vi "calc-total-kinetics.vi"(6 "cluster in":T1={"Kinetics"=[], "Spectrum"=[], "Experiments groups"=[], "GRAPH EXPERIMENTAL DATA"=[], "error out"={"status"=FALSE, "code"=0, "source"=""}, "group"=0, "exp selected"=0, "# exp"=0, "kinetics plot names"=[], "spectra plot names"=[], "FromToWave"={"FromWave"=0.0, "ToWave"=0.0}, "Laser shutter task"="", "Accelerator task"="", "Motor task"="", "GRAPH EXPERIMENTAL DATA ref"=refnum, "timedelays"=[0.0, 0.0, 0.0, 0.0, 0.0, 0.0, 0.0, 0.06019061100911815, 0.0521779104562645, 0.045231877429679615, 0.03921051490799832, 0.033990728811568754, 0.029465811603150715, 0.025543260876973825, 0.02214288834180205, 0.01919518054014414, 0.016639877791965713, 0.014424742312398925, 0.012504490320209958, 0.010839866306230088, 0.009396840537117498, 0.008145913389103785, 0.00706151229029317, 0.006121468943269439, 0.005306566140927374, 0.004600144911132549, 0.003987763959109073, 0.0034569044455719407, 0.00299671406541447, 0.0025977851951783253, 0.0022519625739982996, 0.00195217658646366, 0.0016922987392150965, 0.0014670163768006634, 0.0012717240756200802, 0.0011024294957352762, 0.0009556717658856477, 0.0008284507332614981, 0.0007181656316962257, 0.0006225619144775864, 0.0005396851648867825, 0.00046784114226338394, 0.0004055611468220084, 0.0003515719951773376, 0.00030476999279031153, 0.00026419837125694315, 0.00022902772919263772, 0.0001985390768670671, 0.0001721091379728629, 0.00014919760805372974, 0.00012933610911736794], "wavelengths"=[0.0, 0.0, 0.0, 0.0, 0.0, 0.0, 0.0, 0.06019061100911815, 0.0521779104562645, 0.045231877429679615, 0.03921051490799832, 0.033990728811568754, 0.029465811603150715, 0.025543260876973825, 0.02214288834180205, 0.01919518054014414, 0.016639877791965713, 0.014424742312398925, 0.012504490320209958, 0.010839866306230088, 0.009396840537117498, 0.008145913389103785, 0.00706151229029317, 0.006121468943269439, 0.005306566140927374, 0.004600144911132549, 0.003987763959109073, 0.0034569044455719407, 0.00299671406541447, 0.0025977851951783253, 0.0022519625739982996, 0.00195217658646366, 0.0016922987392150965, 0.0014670163768006634, 0.0012717240756200802, 0.0011024294957352762, 0.0009556717658856477, 0.0008284507332614981, 0.0007181656316962257, 0.0006225619144775864, 0.0005396851648867825, 0.00046784114226338394, 0.0004055611468220084, 0.0003515719951773376, 0.00030476999279031153, 0.00026419837125694315, 0.00022902772919263772, 0.0001985390768670671, 0.0001721091379728629, 0.00014919760805372974, 0.00012933610911736794], "Experiment"=refnum, "Commentaires exp"=refnum, "FromToDelay"={"FromDelay"=0.0, "ToDelay"=0.0}}, 7 "delay0":dbl, 8 "# points":i32, 9 "deltaT":dbl) -> (0 "cluster out":T1={"Kinetics"=[], "Spectrum"=[], "Experiments groups"=[], "GRAPH EXPERIMENTAL DATA"=[], "error out"={"status"=FALSE, "code"=0, "source"=""}, "group"=0, "exp selected"=0, "# exp"=0, "kinetics plot names"=[], "spectra plot names"=[], "FromToWave"={"FromWave"=0.0, "ToWave"=0.0}, "Laser shutter task"="", "Accelerator task"="", "Motor task"="", "GRAPH EXPERIMENTAL DATA ref"=refnum, "timedelays"=[0.0, 0.0, 0.0, 0.0, 0.0, 0.0, 0.0, 0.06019061100911815, 0.0521779104562645, 0.045231877429679615, 0.03921051490799832, 0.033990728811568754, 0.029465811603150715, 0.025543260876973825, 0.02214288834180205, 0.01919518054014414, 0.016639877791965713, 0.014424742312398925, 0.012504490320209958, 0.010839866306230088, 0.009396840537117498, 0.008145913389103785, 0.00706151229029317, 0.006121468943269439, 0.005306566140927374, 0.004600144911132549, 0.003987763959109073, 0.0034569044455719407, 0.00299671406541447, 0.0025977851951783253, 0.0022519625739982996, 0.00195217658646366, 0.0016922987392150965, 0.0014670163768006634, 0.0012717240756200802, 0.0011024294957352762, 0.0009556717658856477, 0.0008284507332614981, 0.0007181656316962257, 0.0006225619144775864, 0.0005396851648867825, 0.00046784114226338394, 0.0004055611468220084, 0.0003515719951773376, 0.00030476999279031153, 0.00026419837125694315, 0.00022902772919263772, 0.0001985390768670671, 0.0001721091379728629, 0.00014919760805372974, 0.00012933610911736794], "wavelengths"=[0.0, 0.0, 0.0, 0.0, 0.0, 0.0, 0.0, 0.06019061100911815, 0.0521779104562645, 0.045231877429679615, 0.03921051490799832, 0.033990728811568754, 0.029465811603150715, 0.025543260876973825, 0.02214288834180205, 0.01919518054014414, 0.016639877791965713, 0.014424742312398925, 0.012504490320209958, 0.010839866306230088, 0.009396840537117498, 0.008145913389103785, 0.00706151229029317, 0.006121468943269439, 0.005306566140927374, 0.004600144911132549, 0.003987763959109073, 0.0034569044455719407, 0.00299671406541447, 0.0025977851951783253, 0.0022519625739982996, 0.00195217658646366, 0.0016922987392150965, 0.0014670163768006634, 0.0012717240756200802, 0.0011024294957352762, 0.0009556717658856477, 0.0008284507332614981, 0.0007181656316962257, 0.0006225619144775864, 0.0005396851648867825, 0.00046784114226338394, 0.0004055611468220084, 0.0003515719951773376, 0.00030476999279031153, 0.00026419837125694315, 0.00022902772919263772, 0.0001985390768670671, 0.0001721091379728629, 0.00014919760805372974, 0.00012933610911736794], "Experiment"=refnum, "Commentaires exp"=refnum, "FromToDelay"={"FromDelay"=0.0, "ToDelay"=0.0}}, 1 "Real delay time, ps":dbl=3790.0, 2 "Kinetics, ps":dbl, 3 "Total, ps":dbl, 5 "# points out":i32)   [LabVIEW 2015]
uses:
  controls/control-cluster.ctl
  Classes/Experiments_group.lvclass
  Classes/Experiment.lvclass
panel:
  in  "y":dbl=9000.0 format="%#_13g"
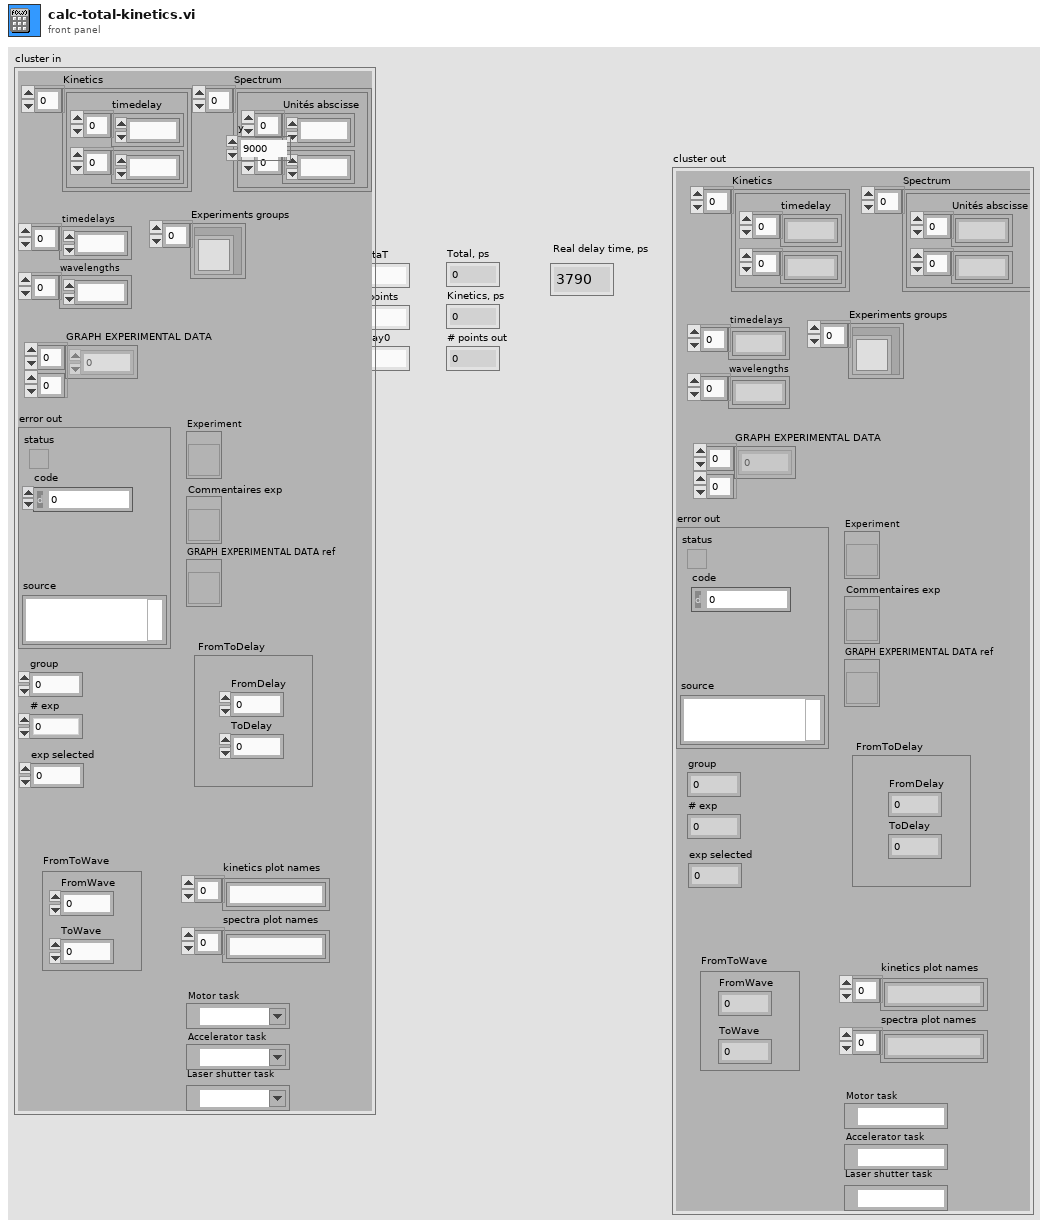
[diagram p1: front panel]
types:
  T1 = typedef "control-cluster.ctl" = cluster{"Kinetics":cluster{"timedelay":dbl[], dbl[]}[], "Spectrum":cluster{"Unités abscisse":dbl[], dbl[]}[], "Experiments groups":refnum<class "Experiments_group.lvclass">[], "GRAPH EXPERIMENTAL DATA":dbl[][], "error out":errorcluster, "group":i32, "exp selected":i32, "# exp":i32, "kinetics plot names":string[], "spectra plot names":string[], "FromToWave":cluster{"FromWave":dbl, "ToWave":dbl}, "Laser shutter task":refnum<k21>, "Accelerator task":refnum<k21>, "Motor task":refnum<k21>, "GRAPH EXPERIMENTAL DATA ref":refnum<vi>, "timedelays":dbl[], "wavelengths":dbl[], "Experiment":refnum<vi>, "Commentaires exp":refnum<vi>, "FromToDelay":cluster{"FromDelay":dbl, "ToDelay":dbl}}
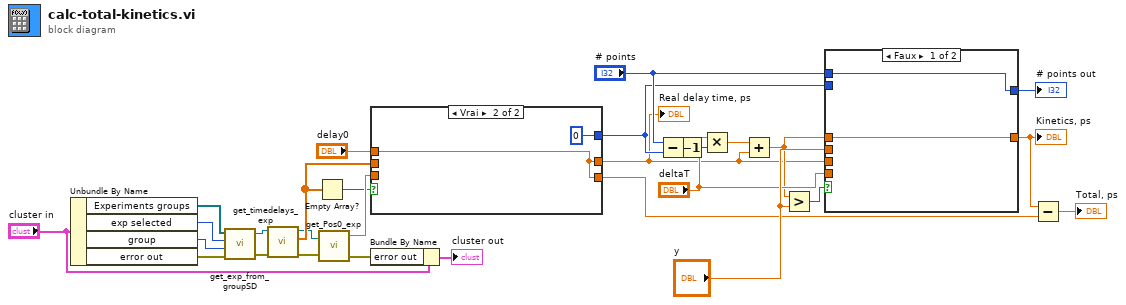
[diagram p0: block diagram]
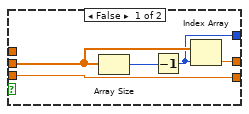
[diagram p2: hidden frame]
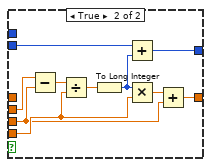
[diagram p3: hidden frame]
diagram:
  n1 = Unbundle By Name("cluster in") -> ("Experiments groups"=w18:refnum<class "Experiments_group.lvclass">[], "exp selected"=w19:i32, "group"=w20:i32, "error out"=w21:errorcluster)
  n2 = call "get_exp_from_groupSD.vi"("error in (no error)"=w21, "group"=w20, "exp selected"=w19, "Experiments groups"=w18) -> ("error out"=w15:errorcluster, "Experiment out"=w16:refnum<class "Experiment.lvclass">)  [unwired: 1 out]
  n3 = call-dynamic "get_timedelays_exp.vi"("error in (no error)"=w15, "Experiment.lvclass in"=w16) -> ("error out"=w12:errorcluster, "timedelays"=w17:dbl[], "Experiment.lvclass out"=w13:refnum<class "Experiment.lvclass">)  [unwired: 7 in]
  n4 = Empty Array?(array=w17) -> (empty?=w5:bool)
  n5 = call-dynamic "get_Pos0_exp.vi"("Experiment.lvclass in"=w13, "error in (no error)"=w12) -> ("Delay0,ps"=w10:dbl, "error out"=w7:errorcluster)  [unwired: 1 out]
  n6 = case shown="Vrai" w5 {
    tunnel: [w34 w35] -> w9
    tunnel: w17 -> [w33 _]
    tunnel: [w30 0 ("x")] -> w14
    tunnel: [w31 w35] -> w3
    tunnel: "delay0" -> [_ w35]
    tunnel: w10 -> [w31 _]
    frame False {
      n7 = Array Size(array=w33) -> (size(s)=w32:i32)
      n8 = Decrement(x=w32) -> (x-1=w30:i32)
      n9 = Index Array(array=w33, index=w30) -> (element=w34:dbl)
    }
    frame True {
    }
  }
  "Real delay time, ps" <- w9
  n10 = Bundle By Name(cluster="cluster in", "error out"=w7) -> (→"cluster out":T1)
  n11 = Subtract(x="# points", y=w14) -> (x-y=w25:i32)
  n12 = Decrement(x=w25) -> (x-1=w1:i32)
  n13 = Multiply(x="deltaT", y=w1) -> (x*y=w24:dbl)
  n14 = Add(x=w24, y=w9) -> (x+y=w22:dbl)
  n15 = Greater?(x=w22, y="y") -> (0:w29:bool)
  n16 = case shown="Faux" w29 {
    tunnel: "y" -> [_ w48]
    tunnel: [w38 w41] -> w27
    tunnel: [w37 w42] -> w2
    tunnel: "deltaT" -> [_ w44]
    tunnel: "# points" -> [w38 _]
    tunnel: w22 -> [w37 _]
    tunnel: w9 -> [_ w43]
    tunnel: w14 -> [_ w39]
    frame False {
    }
    frame True {
      n17 = Subtract(x=w48, y=w43) -> (x-y=w47:dbl)
      n18 = Divide(x=w47, y=w44) -> (x/y=w46:dbl)
      n19 = To Long Integer(number=w46) -> (32bit integer=w40:i32)
      n20 = Add(x=w39, y=w40) -> (x+y=w41:i32)
      n21 = Multiply(x=w40, y=w44) -> (x*y=w45:dbl)
      n22 = Add(x=w45, y=w43) -> (x+y=w42:dbl)
    }
  }
  "Kinetics, ps" <- w2
  "# points out" <- w27
  n23 = Subtract(x=w2, y=w3) -> (x-y=→"Total, ps":dbl)
